vi "_Create.vi"(8 "error in (no error)":errorcluster) -> (0 "error out":errorcluster, 3 "StopSignal":T1)   [LabVIEW 2017, in "StopSignal.lvlib"]
uses:
  StopSignal.lvlib
  Typedef/StopSignal.ctl
  Typedef/Def-StopSignalData.ctl
  Typedef/def-StopReason.ctl
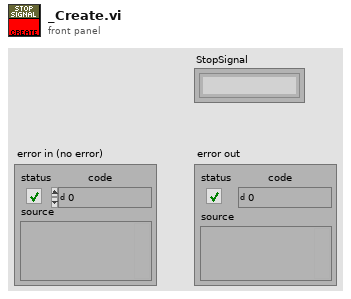
[diagram p1: front panel]
types:
  T1 = typedef "StopSignal.lvlib/StopSignal.ctl" = refnum<k1>
  T2 = typedef "StopSignal.lvlib/def-StopReason.ctl" = cluster{"Reason":string, "timestamp":timestamp}
  T3 = typedef "StopSignal.lvlib/Def-StopSignalData.ctl" = cluster{"StopEvent":refnum<user-event>, "StopNotifier":refnum<notifier>, "StopReason":T2}
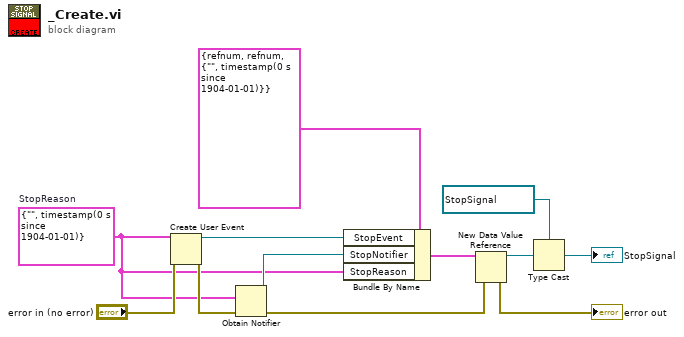
[diagram p0: block diagram]
diagram:
  w1 = T2 {"Reason"="", "timestamp"=timestamp(0 s since 1904-01-01)}  # StopReason
  w7 = T1 refnum items=["StopSignal"] ("StopSignal")
  n1 = Create User Event(user event datatype=w1, error in="error in (no error)") -> (user event=w11:refnum<user-event>, error out=w4:errorcluster)
  n2 = Obtain Notifier(notification data type=w1, error in (no error)=w4) -> (notifier out=w10:refnum<notifier>, error out=w2:errorcluster)  [unwired: 2 in, 1 out]
  n3 = Bundle By Name(cluster=T3 {"StopEvent"=refnum, "StopNotifier"=refnum, "StopReason"={"Reason"="", "timestamp"=timestamp(0 s since 1904-01-01)}} ("Def-xxxxx"), "StopEvent"=w11, "StopNotifier"=w10, "StopReason"=w1) -> (w9:T3)
  n4 = New Data Value Reference(data value=w9, error in=w2) -> (data value reference=w8:refnum<data-value>, error out=→"error out":errorcluster)
  n5 = Type Cast(type=w7, x=w8) -> (*(type *) &x=→"StopSignal":T1)
